vi "保存成mat文件.vi"(0 "数组":dbl[][](array[numeric])) -> ()   [LabVIEW 2014]
panel:
  out "转置的数组":dbl[][](array[numeric])
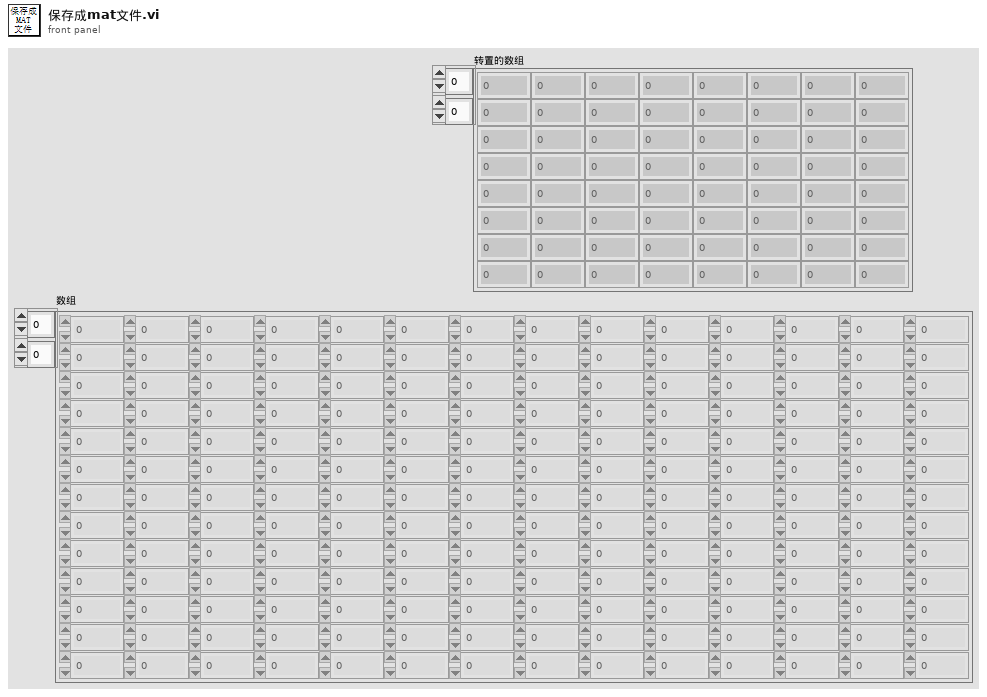
[diagram p1: front panel]
types:
  T1 = enum16{"open", "replace", "create", "open or create", "replace or create", "replace or create with confirmation"}
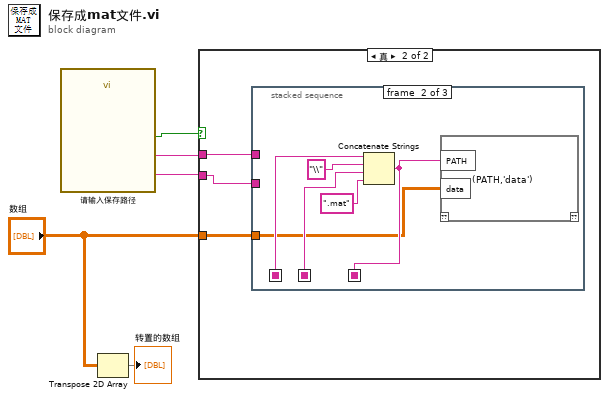
[diagram p0: block diagram]
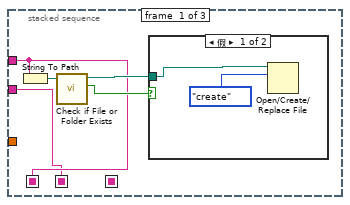
[diagram p3: hidden frame]
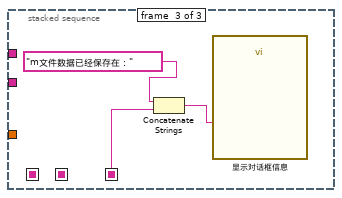
[diagram p5: hidden frame]
diagram:
  n1 = call "请输入保存路径"() -> ("请输入文件名称"=w3:string, "请输入保存路径"=w4:string, "确定"=w5:bool)  [unwired: 16 in, 1 out]
  n2 = Transpose 2D Array(2D array="数组") -> (transposed array=→"转置的数组":dbl[][])
  n3 = case shown="真" w5 {
    tunnel: w4 -> [_ w8]
    tunnel: w3 -> [_ w7]
    tunnel: "数组" -> [_ w6]
    frame False {
    }
    frame True {
      n4 = stacked-sequence {
        seq-local: [w10 _ _] -> [_ w21 _]
        seq-local: [w9 _ _] -> [_ w19 _]
        seq-local: [_ w17 _] -> [_ _ w23]
        tunnel: w8 -> [w10 _ _]
        tunnel: w7 -> [w9 _ _]
        tunnel: w6 -> [_ w16 _]
        frame #0 {
          n5 = String To Path(string=w10) -> (path=w13:path)
          n6 = call <vilib>:"Check if File or Folder Exists.vi"("path"=w13) -> ("file or folder exists?"=w12:bool, "dup path"=w11:path)  [unwired: 8 in, 1 out]
          n7 = case shown="假" w12 {
            tunnel: w11 -> [w14 _]
            frame False {
              n8 = Open/Create/Replace File(file path (use dialog)=w14, operation (0:open)=T1."create" ("操作(0:open)")) -> ()  [unwired: 4 in, 3 out]
            }
            frame True {
            }
          }
        }
        frame #1 {
          n9 = Concatenate Strings(w21, "\\", w19, ".mat") -> (w17:string)
          n10 = script code="save(PATH,'data')"("PATH"=w17, "data"=w16) -> ()  [unwired: 1 in, 1 out]
        }
        frame #2 {
          n11 = Concatenate Strings("m文件数据已经保存在：" ("字符串"), w23) -> (w22:string)
          n12 = call "显示对话框信息"("Message"=w22) -> ()  [unwired: 9 in, 2 out]
        }
      }
    }
  }
